vi "BufferSequence.vi"() -> (2 "NumPoints":i32, 3 "Sequencing error":bool)   [LabVIEW 2011]
uses:
  <vilib>/rvi/DataTransferAndStorage/Container/Common/niFpgaContainerExecOnDevCompGetState.vi
  <vilib>/rvi/FIFO/Fifo_Resource/nirvififoEmulationSetSize.vi
  <vilib>/rvi/DataTransferAndStorage/Container/Common/niFpgaContainerGetUniqueNameForEmu.vi
  <vilib>/rvi/interface/RandomDataEmulation/nirviRandomDataFPGAFIFO.vi
  <vilib>/rvi/interface/RandomDataEmulation/niFpgaRandomDataHandleErrors.vi
  <vilib>/rvi/eio/common/nirviEmuReportErrorAndStop.vi
  <vilib>/rvi/DataTransferAndStorage/Container/XNode/niFpgaContainer.xnode
  <vilib>/rvi/FIFO/Fifo_Resource/niFpgaFifoEmulationRefIn.vi
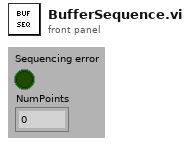
[diagram p1: front panel]
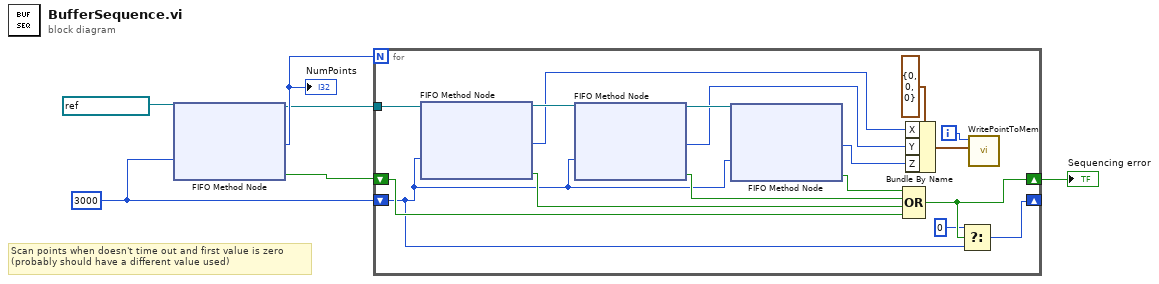
[diagram p0: block diagram]
diagram:
  w6 = 3000 ("Timeout")
  # "Scan points when doesn't time out and first value is zero \n(probably should have a different value used)"
  n1 = xnode ("FIFO Method Node")("Timeout"=w6, "FIFO In"=refnum<k21> "Coordinate") -> ("Element"=w3:i32, "Timed Out?"=w1:bool, "FIFO Out"=w2:refnum<k21>)
  "NumPoints" <- w3
  n2 = for {
    N: w3 -> [_]
    shift-right: [w9] -> w4
    shift-left: w1 -> [w22]
    tunnel: w2 -> [w21]
    shift-right: [w10] -> _
    shift-left: w6 -> [w7]
    i -> [w11]
    n3 = xnode ("FIFO Method Node")("Timeout"=w7, "FIFO In"=w21) -> ("Element"=w13:i32, "Timed Out?"=w23:bool, "FIFO Out"=w20:refnum<k21>)
    n4 = xnode ("FIFO Method Node")("Timeout"=w7, "FIFO In"=w20) -> ("Element"=w14:i32, "Timed Out?"=w18:bool, "FIFO Out"=w19:refnum<k21>)
    n5 = xnode ("FIFO Method Node")("Timeout"=w7, "FIFO In"=w19) -> ("Element"=w15:i32, "Timed Out?"=w17:bool)  [unwired: 1 out]
    n6 = Compound Arithmetic op=OR(w17, w18, w23, w22) -> (w9:bool)
    n7 = Bundle By Name(cluster=cluster{"X":i32, "Y":i32, "Z":i32} {"X"=0, "Y"=0, "Z"=0} ("Point"), "X"=w13, "Y"=w14, "Z"=w15) -> (w12:cluster{"X":i32, "Y":i32, "Z":i32})
    n8 = Select(t=u32 0, s=w9, f=w7) -> (s? t:f=w10:u32)
    n9 = call "WritePointToMem.vi"("Point"=w12, "PointNum"=w11) -> ()  [unwired: 10 in]
  }
  "Sequencing error" <- w4
